vi "LAbo2.3.2.vi"() -> ()   [LabVIEW 2020]
panel:
  out "x2:":string
  out "x1:":string
  out "ile jest pierwiastkow trojmianu kwadratowego:":string
  in  "Wartość c:":dbl
  in  "Wartość b:":dbl
  in  "Wartość a:":dbl
  out "wzór ogólny:":string
  out "Opis działania programu:":string caption="Opis działania programu"
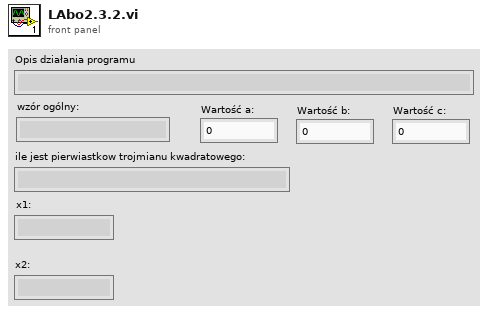
[diagram p1: front panel]
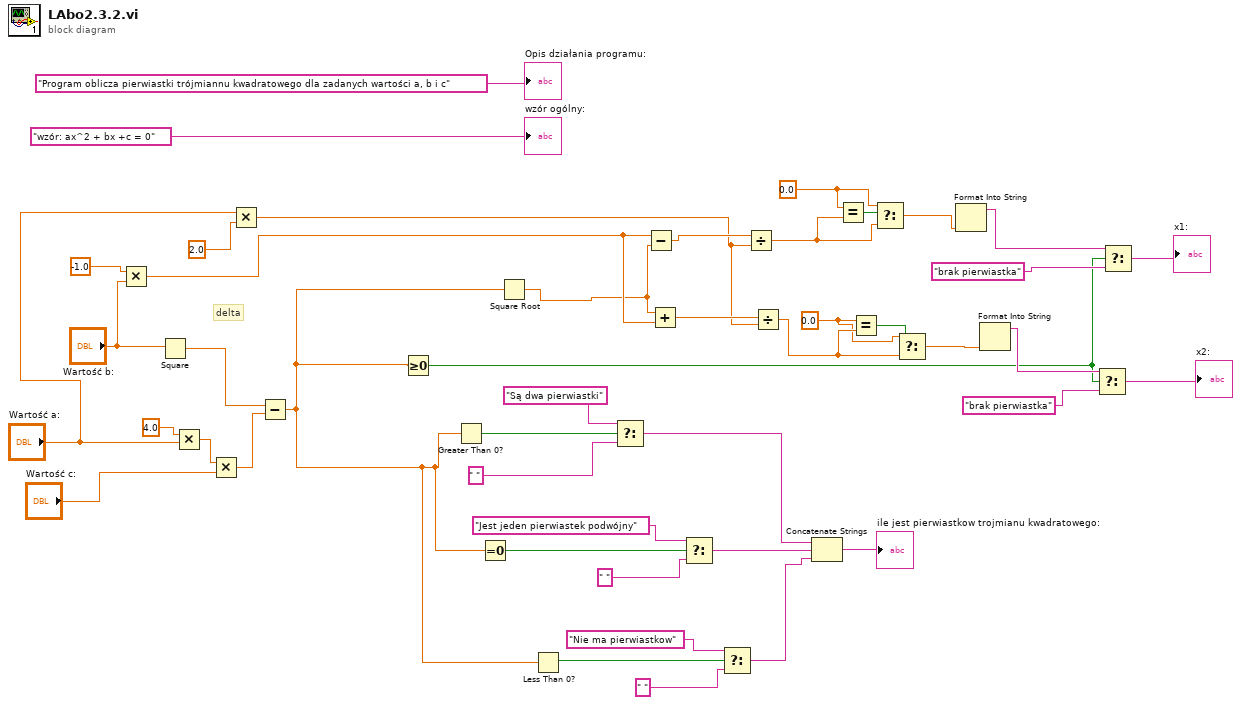
[diagram p0: block diagram]
diagram:
  w1 = 0.0
  w2 = 0.0
  # "delta"
  n1 = Multiply(x=-1.0, y="Wartość b:") -> (x*y=w23:dbl)
  n2 = Square(x="Wartość b:") -> (x^2=w27:dbl)
  n3 = Multiply(x=4.0, y="Wartość a:") -> (x*y=w41:dbl)
  n4 = Multiply(x=w41, y="Wartość c:") -> (x*y=w40:dbl)
  n5 = Multiply(x="Wartość a:", y=2.0) -> (x*y=w18:dbl)
  n6 = Subtract(x=w27, y=w40) -> (x-y=w9:dbl)
  n7 = Greater Or Equal To 0?(x=w9) -> (x >= 0?=w10:bool)
  n8 = Greater Than 0?(x=w9) -> (x > 0?=w26:bool)
  n9 = Equal To 0?(x=w9) -> (x = 0?=w37:bool)
  n10 = Square Root(x=w9) -> (sqrt(x)=w17:dbl)
  n11 = Less Than 0?(x=w9) -> (x < 0?=w32:bool)
  n12 = Select(t="Są dwa pierwiastki", s=w26, f=" ") -> (s? t:f=w28:string)
  n13 = Subtract(x=w23, y=w17) -> (x-y=w20:dbl)
  n14 = Add(x=w17, y=w23) -> (x+y=w19:dbl)
  n15 = Select(t="Jest jeden pierwiastek podwójny", s=w37, f=" ") -> (s? t:f=w31:string)
  n16 = Select(t="Nie ma pierwiastkow", s=w32, f=" ") -> (s? t:f=w30:string)
  n17 = Divide(x=w20, y=w18) -> (x/y=w7:dbl)
  n18 = Divide(x=w19, y=w18) -> (x/y=w3:dbl)
  n19 = Concatenate Strings(w28, w31, w30) -> (→"ile jest pierwiastkow trojmianu kwadratowego:":string)
  n20 = Equal?(x=w2, y=w7) -> (x = y?=w8:bool)
  n21 = Equal?(x=w1, y=w3) -> (x = y?=w5:bool)
  n22 = Select(t=w2, s=w8, f=w7) -> (s? t:f=w6:dbl)
  n23 = Select(t=w1, s=w5, f=w3) -> (s? t:f=w4:dbl)
  n24 = Format Into String(w6) -> (resulting string=w15:string)  [unwired: 3 in, 1 out]
  n25 = Format Into String(w4) -> (resulting string=w12:string)  [unwired: 3 in, 1 out]
  n26 = Select(t=w12, s=w10, f="brak pierwiastka") -> (s? t:f=→"x2:":string)
  n27 = Select(t=w15, s=w10, f="brak pierwiastka") -> (s? t:f=→"x1:":string)
  "Opis działania programu:" <- "Program oblicza pierwiastki trójmiannu kwadratowego dla zadanych wartości a, b i c"
  "wzór ogólny:" <- "wzór: ax^2 + bx +c = 0"
